vi "plate_pwm.vi"(11 "period (ms)":u32=16) -> ()   [LabVIEW 2015]
panel:
  out "Waveform Chart":i16(graph)
  out "pwm":dbl min=0.0 max=100.0 step=1.0
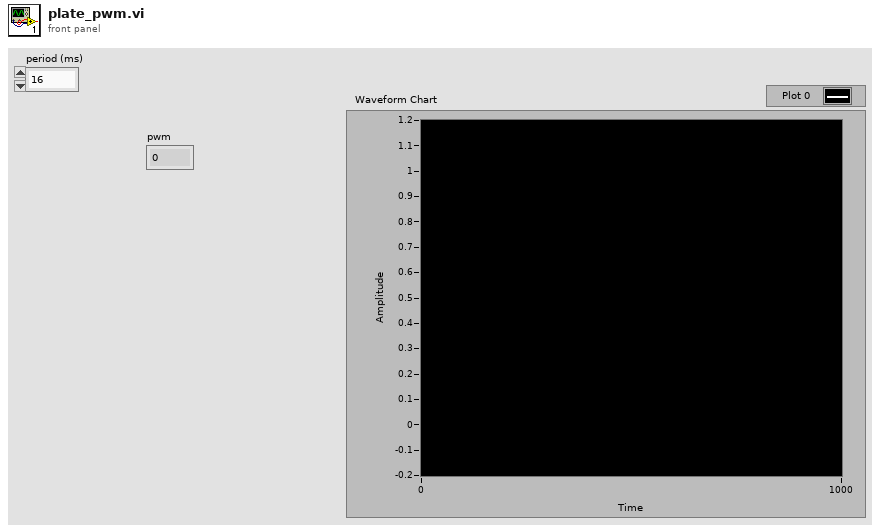
[diagram p1: front panel]
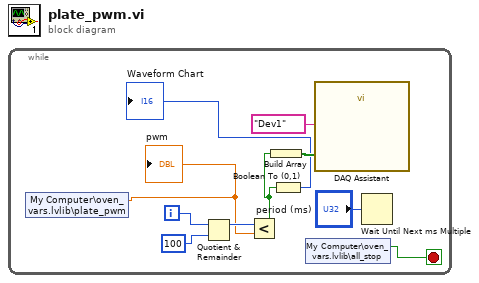
[diagram p0: block diagram]
diagram:
  n1 = while {
    i -> [w10]
    stop <- w1 stop-if-true
    n2 = shared-variable "My Computer\\oven_vars.lvlib\\plate_pwm"() -> (w2:dbl)  [unwired: 1 in, 1 out]
    "pwm" <- w2
    n3 = Quotient & Remainder(x=w10, y=100) -> (x-y*floor(x/y)=w8:i32)  [unwired: 1 out]
    n4 = Less?(x=w8, y=w2) -> (x < y?=w6:bool)
    n5 = Build Array(w6) -> (w7:bool[])
    n6 = Boolean To (0,1)(Boolean=w6) -> (0, 1=→"Waveform Chart":i16)
    n7 = shared-variable "My Computer\\oven_vars.lvlib\\all_stop"() -> (w1:bool)  [unwired: 1 in, 1 out]
    n8 = call "DAQ Assistant"("data"=w7, "device name"=tag "Dev1") -> ()  [unwired: 16 in, 2 out]
    n9 = Wait Until Next ms Multiple(millisecond multiple="period (ms)") -> ()  [unwired: 1 out]
  }
